vi "TCP_联机.vi"(7 "写入地址":u32=1000, 9 "写入数据":i8, 11 "联机":bool) -> ()   [LabVIEW 2013]
uses:
  S7Ref.vi
panel:
  in  "error in (no error)":errorcluster
  out "error out":errorcluster
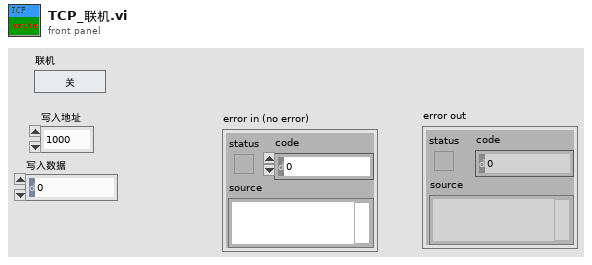
[diagram p1: front panel]
types:
  T1 = cluster{"Boolean array[0]":bool, "Boolean array[1]":bool, "Boolean array[2]":bool, "Boolean array[3]":bool, "Boolean array[4]":bool, "Boolean array[5]":bool, "Boolean array[6]":bool, "Boolean array[7]":bool}
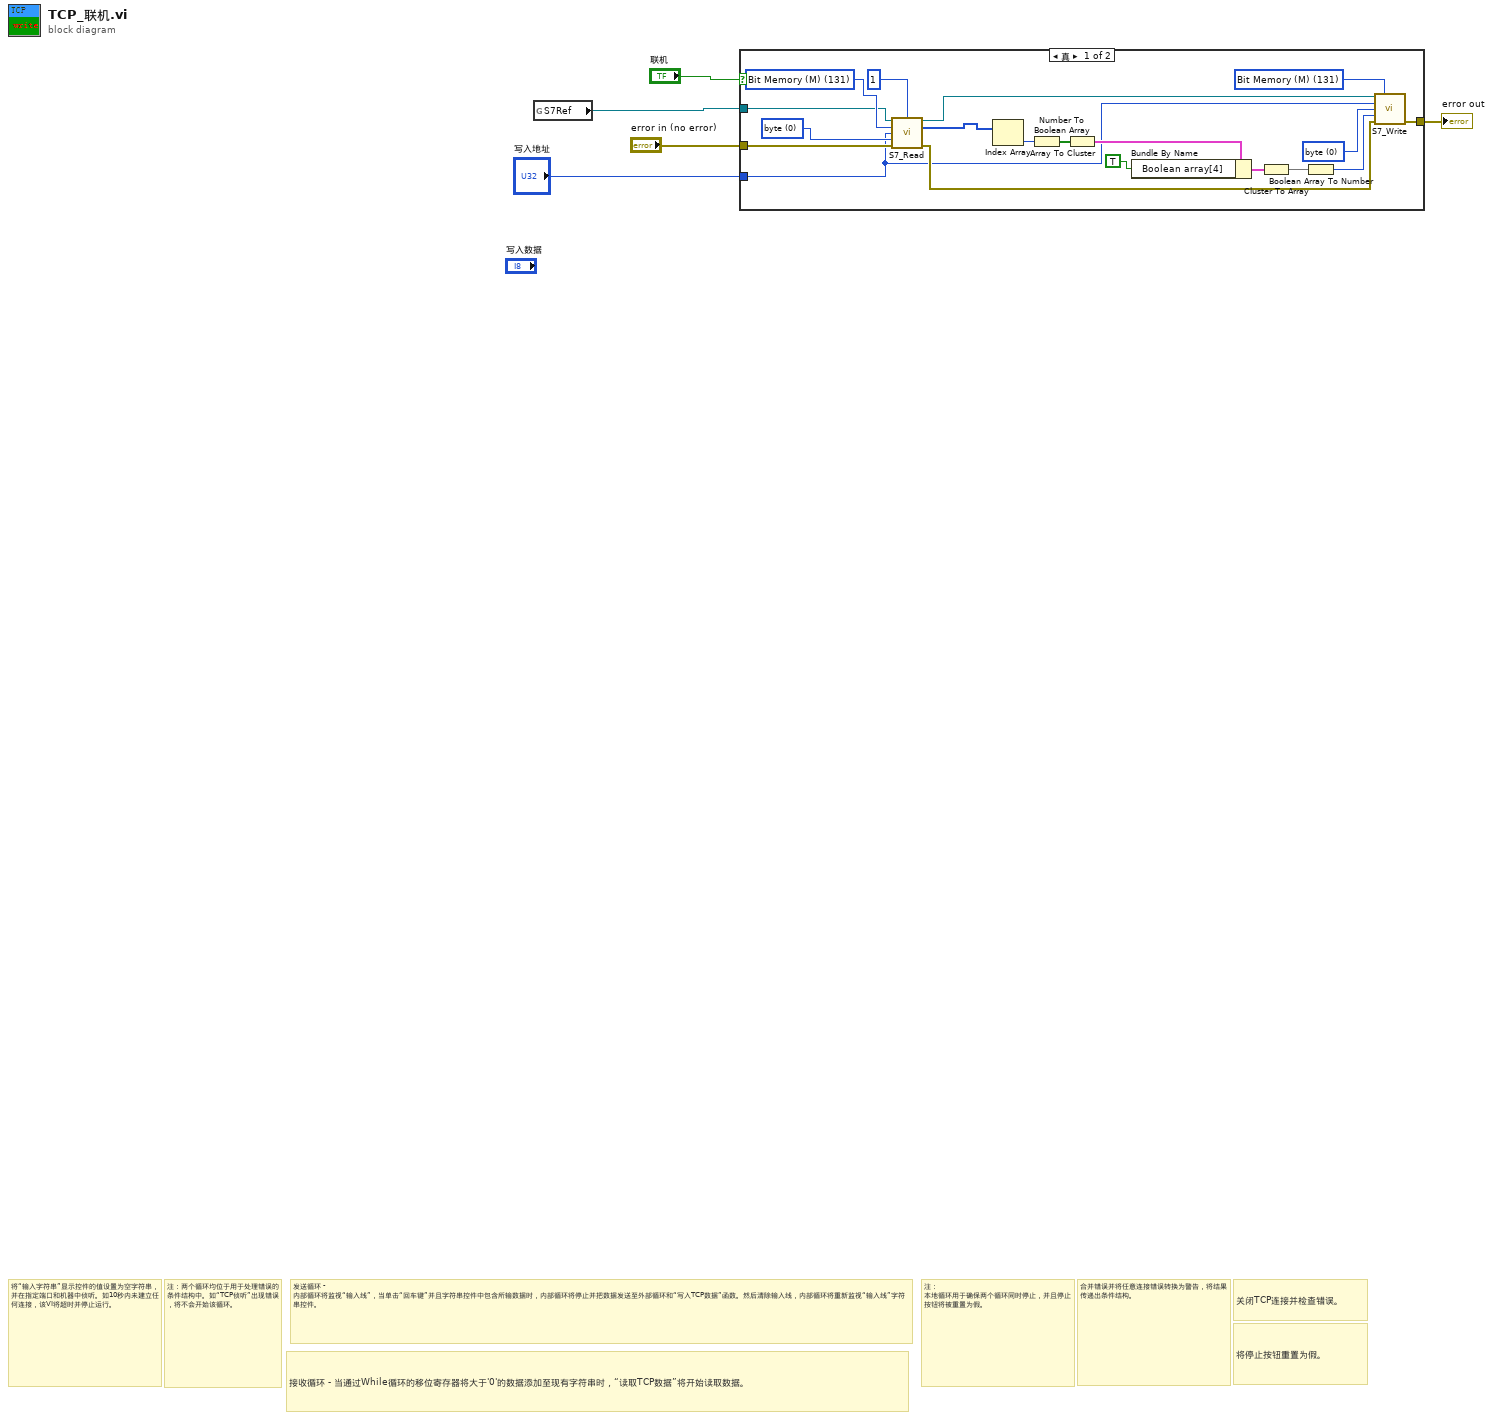
[diagram p0: block diagram]
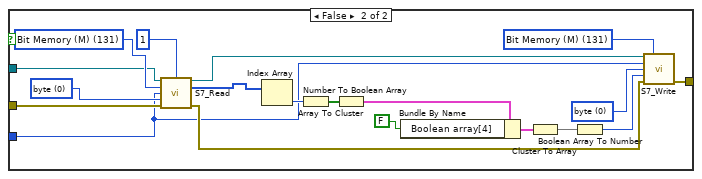
[diagram p2: hidden frame]
diagram:
  # "将停止按钮重置为假。"
  # "关闭TCP连接并检查错误。"
  # "注：两个循环均位于用于处理错误的条件结构中。如“TCP侦听”出现错误，将不会开始该循环。"
  # "合并错误并将任意连接错误转换为警告，将结果传递出条件结构。"
  # "注： 本地循环用于确保两个循环同时停止，并且停止按钮将被重置为假。"
  # "接收循环 - 当通过While循环的移位寄存器将大于'0'的数据添加至现有字符串时，“读取TCP数据”将开始读取数据。"
  # "发送循环 - 内部循环将监视“输入线”，当单击“回车键”并且字符串控件中包含所输数据时，内部循环将停止并把数据发送至外部循环和“写入TCP数据”函数。然后清除输入线，内部循环将重新监视“输入线”字符串控件。"
  # "将“输入字符串”显示控件的值设置为空字符串，并在指定端口和机器中侦听。如10秒内未建立任何连接，该VI将超时并停止运行。"
  n1 = global read "S7Ref.vi" "S7Ref"() -> (w3:refnum<k5>)
  n2 = case shown="真" "联机" {
    tunnel: "error in (no error)" -> [w11 w30]
    tunnel: w3 -> [w9 w28]
    tunnel: "写入地址" -> [w6 w25]
    tunnel: [w7 w26] -> w1
    frame True {
      w16 = u16 0 items=["byte", "word", "Dword"] ("数据类型")
      w14 = u8 131 items=["I/O (P)"=128, "Input (I)"=129, "Output (Q)"=130, "Bit Memory (M)"=131, "Data (DB)"=132, "Instance Data (DI)"=133, "Local Data (L)"=134, "Predecessor Local Data (VL)"=135] ("寄存器类型")
      w12 = u16 0 items=["byte", "word", "Dword"] ("数据类型")
      w13 = u8 131 items=["I/O (P)"=128, "Input (I)"=129, "Output (Q)"=130, "Bit Memory (M)"=131, "Data (DB)"=132, "Instance Data (DI)"=133, "Local Data (L)"=134, "Predecessor Local Data (VL)"=135] ("寄存器类型")
      n3 = call "S7_Read .vi"("TCP"=w9, "读取长度"=u16 1, "寄存器类型"=w14, "起始地址"=w6, "数据类型"=w16, "error in"=w11) -> ("TCP"=w8:refnum<k5>, "数据"=w10:u32[], "error out"=w24:errorcluster)  [unwired: 6 in, 1 out]
      n4 = Index Array(array=w10) -> (element=w19:u32)  [unwired: 1 in]
      n5 = Number To Boolean Array(number=w19) -> (Boolean array=w18:bool[])
      n6 = Array To Cluster(array=w18) -> (cluster=w20:T1)
      n7 = Bundle By Name(cluster=w20, "Boolean array[4]"=TRUE) -> (w22:T1)
      n8 = Cluster To Array(cluster=w22) -> (array=w21:bool[])
      n9 = Boolean Array To Number(Boolean array=w21) -> (number=w23:u32)
      n10 = call "S7_Write .vi"("TCP"=w8, "寄存器类型"=w13, "写入地址"=w6, "数据类型"=w12, "写入数据"=w23, "error in"=w24) -> ("error out"=w7:errorcluster)  [unwired: 7 in, 2 out]
    }
    frame False {
      w35 = u16 0 items=["byte", "word", "Dword"] ("数据类型")
      w33 = u8 131 items=["I/O (P)"=128, "Input (I)"=129, "Output (Q)"=130, "Bit Memory (M)"=131, "Data (DB)"=132, "Instance Data (DI)"=133, "Local Data (L)"=134, "Predecessor Local Data (VL)"=135] ("寄存器类型")
      w31 = u16 0 items=["byte", "word", "Dword"] ("数据类型")
      w32 = u8 131 items=["I/O (P)"=128, "Input (I)"=129, "Output (Q)"=130, "Bit Memory (M)"=131, "Data (DB)"=132, "Instance Data (DI)"=133, "Local Data (L)"=134, "Predecessor Local Data (VL)"=135] ("寄存器类型")
      n11 = call "S7_Read .vi"("TCP"=w28, "读取长度"=u16 1, "寄存器类型"=w33, "起始地址"=w25, "数据类型"=w35, "error in"=w30) -> ("TCP"=w27:refnum<k5>, "数据"=w29:u32[], "error out"=w43:errorcluster)  [unwired: 6 in, 1 out]
      n12 = Index Array(array=w29) -> (element=w38:u32)  [unwired: 1 in]
      n13 = Number To Boolean Array(number=w38) -> (Boolean array=w37:bool[])
      n14 = Array To Cluster(array=w37) -> (cluster=w39:T1)
      n15 = Bundle By Name(cluster=w39, "Boolean array[4]"=FALSE) -> (w41:T1)
      n16 = Cluster To Array(cluster=w41) -> (array=w40:bool[])
      n17 = Boolean Array To Number(Boolean array=w40) -> (number=w42:u32)
      n18 = call "S7_Write .vi"("TCP"=w27, "寄存器类型"=w32, "写入地址"=w25, "数据类型"=w31, "写入数据"=w42, "error in"=w43) -> ("error out"=w26:errorcluster)  [unwired: 7 in, 2 out]
    }
  }
  "error out" <- w1
